vi "Relay test.vi"() -> ()   [LabVIEW 2021]
uses:
  ELAN/enums/main_prog_state.ctl
  ELAN/enums/init_state.ctl
  Master CR.lvclass
  Param/TCP Param/TCP Param.lvclass
  D:/my_projects/projects/21/Master CR/Param/Param.lvclass
  Master CR.lvclass/Master CR.ctl
  Param/Param.lvclass/Param.ctl
  Param/TCP Param/TCP Param.lvclass/TCP Param.ctl
  <vilib>/Platform/TimedLoop/XDataNode/timing_clust.ctl
  <vilib>/Platform/TimedLoop/XDataNode/nitl_modes.ctl
  <vilib>/Platform/TimedLoop/XDataNode/wakeup.ctl
  ELAN/enums/close_state.ctl
  Data/Data Model/Read Data Model.vi
  <vilib>/Utility/config.llb/Read Key (String).vi
  <vilib>/Utility/config.llb/Write Key (String).vi
  <vilib>/Platform/TimedLoop/XDataNode/XDataNode.xnode
  Modbus_v121c/Data Model/Device Data Model.lvclass
  <vilib>/Platform/TimedLoop/XDataNode/XDNodeRunTimeDep.lvlib
  ELAN/enums/Param_MB test.lvlib
  Param/Param.lvclass
  <vilib>/Utility/config.llb/NI_LVConfig.lvlib
panel:
  out "N2":u64
  out "N1":u64
  in  "Write":bool
  in  "Read":bool
  out "connects":bool[](array[boolean])
  out "DI":bool[](array[boolean])
  in  "DO":bool[](array[boolean])
  in  "AOint":u16[](array[numeric])
  out "comm error":errorcluster
  out "initialise error":errorcluster
  in  "EP_on":bool
  in  "tick":i64=1000 caption="Время цикла основной программы" min=5 max=2000 step=1
  in  "stop":bool
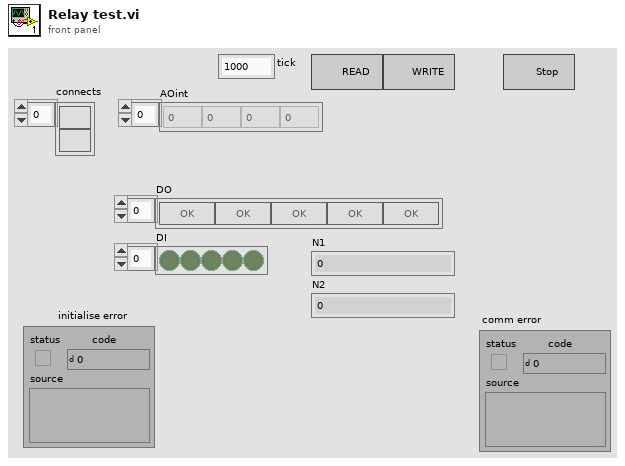
[diagram p1: front panel]
types:
  T1 = cluster{"conn_timeout":i32, "reconn_timeout":i32, "N attempt max":i32, "t_reset_TTL":i32, "write_timeout":i32, "read_timeout":i32, "period":i32}[]
  T2 = cluster{"Remote IP Address":string, "Remote Port":u16}[]
  T3 = typedef "Param_MB test.lvlib/init_state.ctl" = enum16{"Init Data", "Init TMPs", "Init system DB", "Init data DB", "Read Enums", "Init arrays", "Init KFM", "Init Param", "Init AI param", "Init DI param", "Init AO param", "Init DO param", "Init ALR param", "Init save progs", "Read OPC param", "Init Shared Variables", "Init regulators", "Init heaters", "Init Y defs", "Exit"}
  T4 = typedef "Param_MB test.lvlib/main_prog_state.ctl" = enum16{"Read_AI_Param", "Read_DI_Param", "Read_AO_Param", "Read_DO_Param", "Read_ALR_ON_OFF", "Read_ALR_Param", "Read_Param", "Read_REG_Param", "Timers", "AI", "DI", "SendAItoScada", "SendDItoScada", "Alarms", "SendAItoDB", "SendDItoDB", "SendALRtoDB", "Messages", "Controls", "Control HT1", "QN_control", "QN", "QN_state", "Control EB3", "Outputs", "Exit"}
  T5 = cluster{"KFM":string[], "PAR":string[], "AI":string[], "DI":string[], "DI_fast":string[], "AO":string[], "Regs":string[], "DO":string[], "ALR":string[], "System":string[]}
  T6 = typedef "NI_LVConfig.lvlib/Config Data RefNum.ctl" = refnum<k1>
  T7 = cluster{"Enums":cluster{"KFM":string[], "PAR":string[], "AI":string[], "DI":string[], "DI_fast":string[], "AO":string[], "Regs":string[], "DO":string[], "ALR":string[], "System":string[]}, "MBs":refnum<class "Master CR.lvclass">[], "N":string[]}
  T8 = cluster{"current time":timestamp, "Timer_1s":bool, "Timer_10s":bool, "Timer_1day":bool}
  T9 = typedef "XDNodeRunTimeDep.lvlib/timing_clust.ctl" = cluster{"Expected End [f-1]":u64, "Actual End [f-1]":u64, "Finished Late? [f-1]":bool, "Expected End [i-1]":u64, "Actual End [i-1]":u64, "Finished Late? [i-1]":bool, "Expected Start [i]":u64, "Actual Start [i]":u64, "Expected Start [f]":u64, "Actual Start [f]":u64, "Source Name":string, "Structure Name":string, "Period":i64, "Deadline":i64, "Offset":i64, "Start":i64, "Priority":i32, "Timeout":i32, "Mode":T10, "Wakeup Reason":T11, "Error":errorcluster, "Source Type":string, "Secondary Source Type":string, "Global End Time":u64, "Global Start Time":u64, "Frame Duration":u64, "Iteration Duration":u64, "Assigned CPU":i32, "I/O Scan Engine Mode":u32}
  T10 = typedef "XDNodeRunTimeDep.lvlib/nitl_modes.ctl" = enum32{"No Change", "Process missed periods, maintain original phase", "Discard missed periods, maintain original phase", "Process missed periods, ignore original phase", "Discard missed periods, ignore original phase"}
  T11 = typedef "XDNodeRunTimeDep.lvlib/wakeup.ctl" = enum32{"Normal", "Aborted", "Asynchronous wakeup", "Timing source error", "Timed loop error", "Timeout"}
  T12 = typedef "Param_MB test.lvlib/close_state.ctl" = enum16{"QN_state notifier", "QN_control_queue", "ALR notifires", "ALR", "DO notifires", "DO", "AO notifires", "AO", "DI notifres", "DI", "AI notifires", "AI", "OPC", "Param", "SaveMessageProg", "KFM DadaRef", "KFM Registers", "KFM StatusRef", "Exit"}
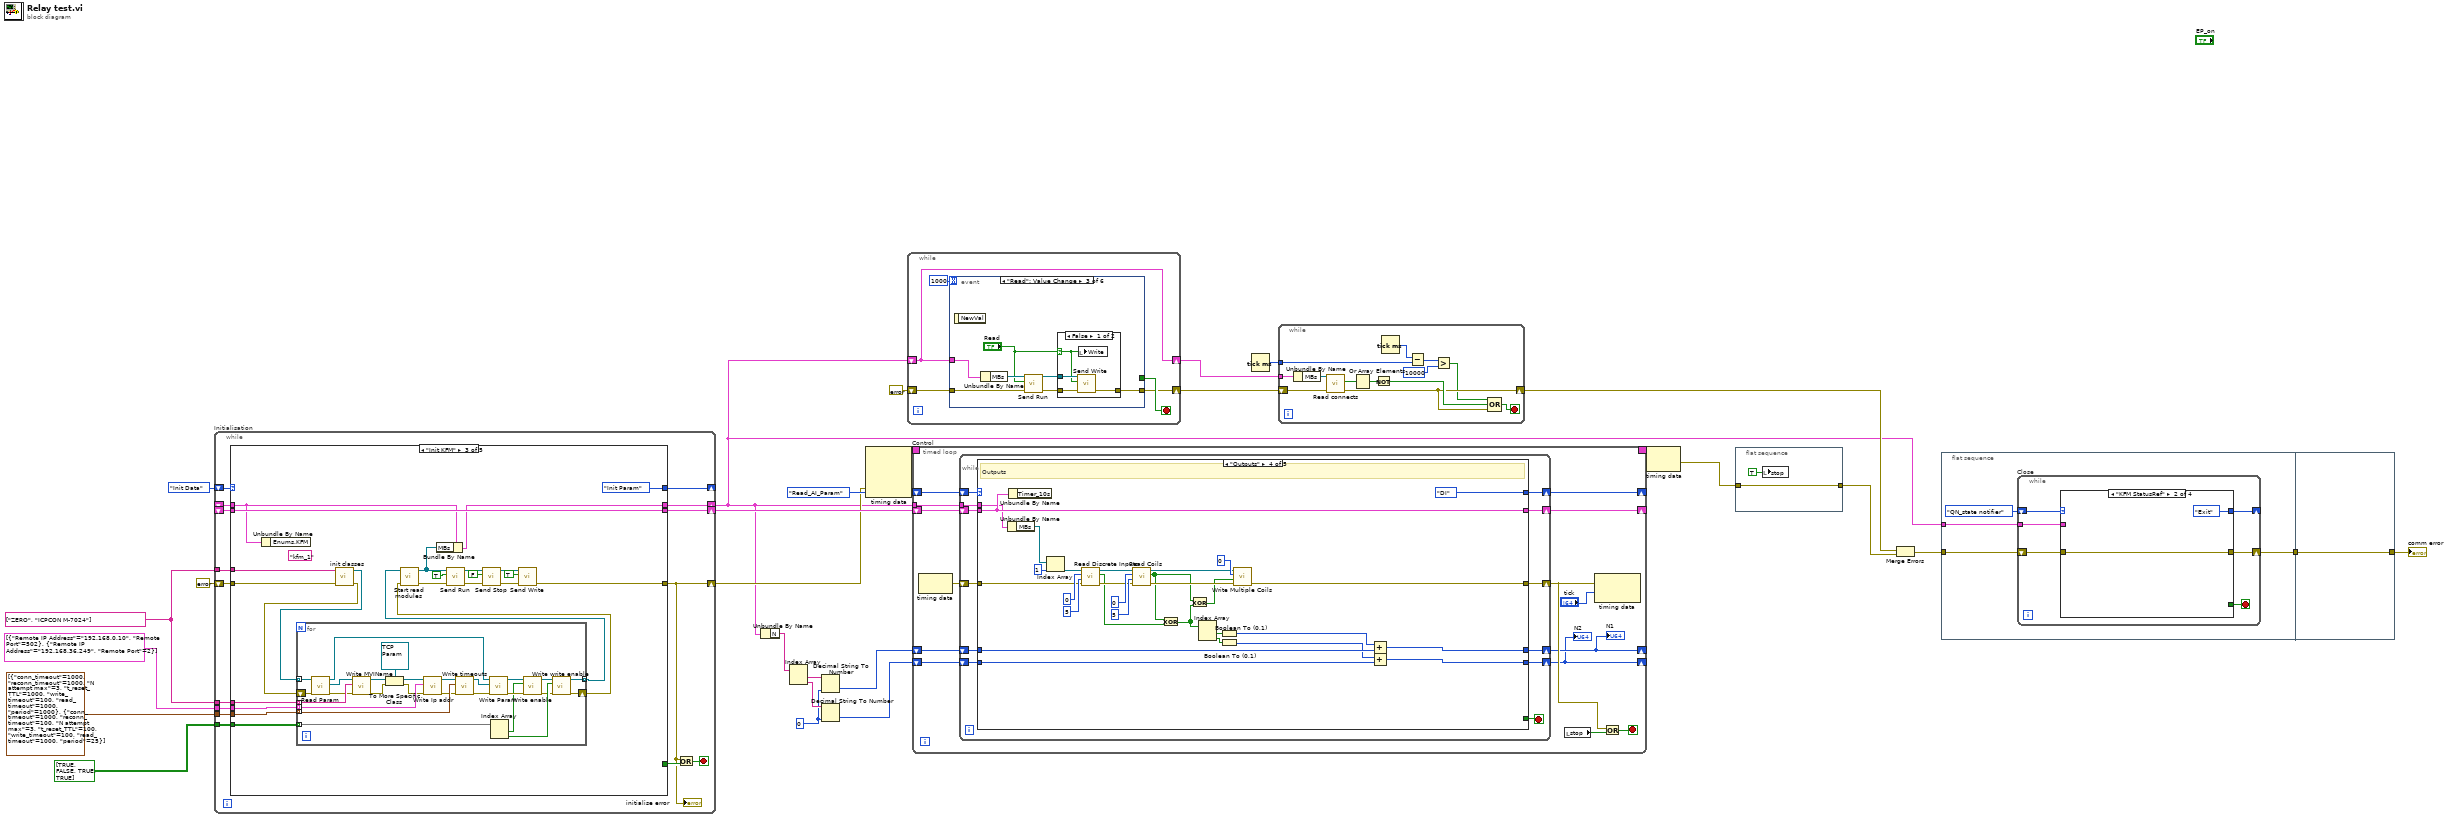
[diagram p0: block diagram]
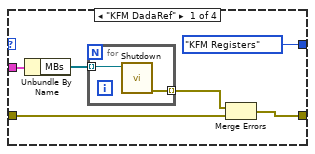
[diagram p2: hidden frame]
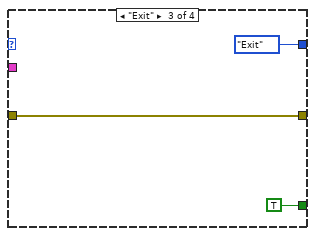
[diagram p3: hidden frame]
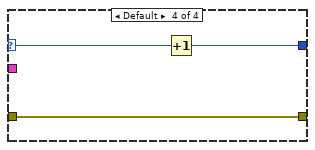
[diagram p4: hidden frame]
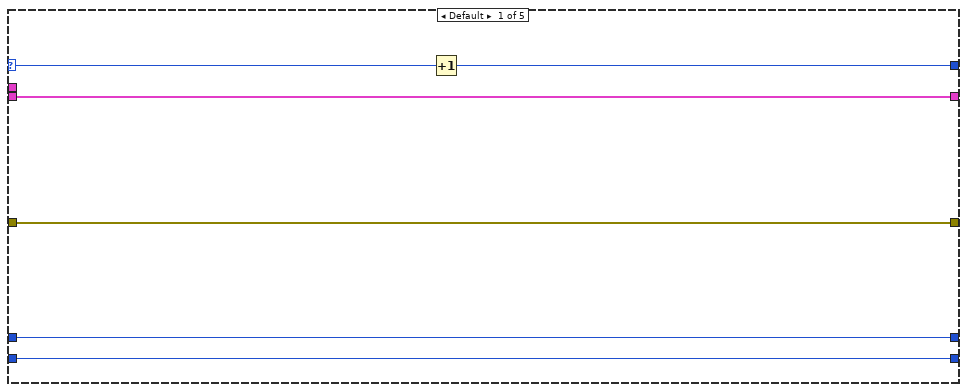
[diagram p5: hidden frame]
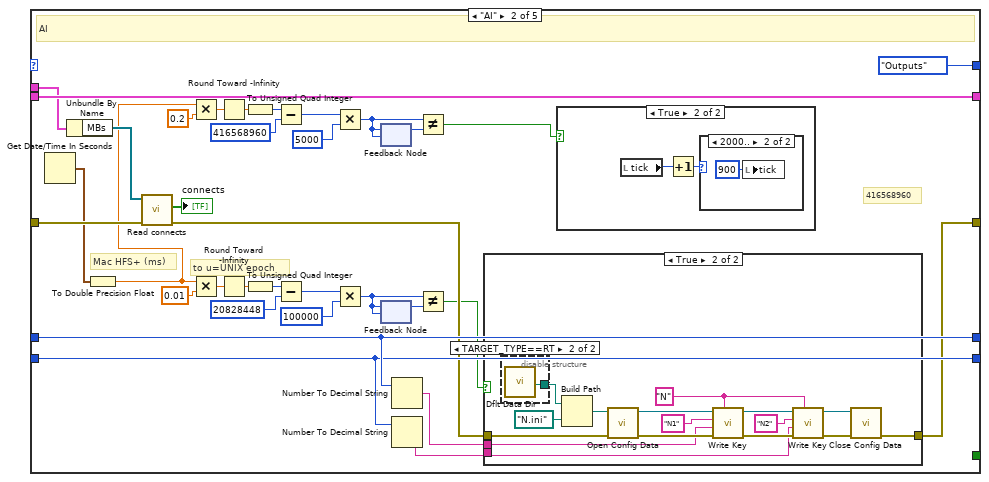
[diagram p6: hidden frame]
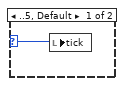
[diagram p8: hidden frame]
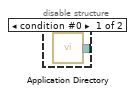
[diagram p10: hidden frame]
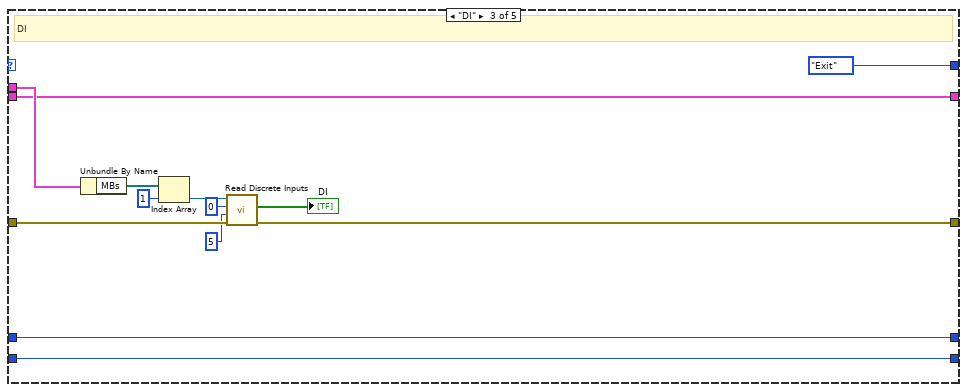
[diagram p11: hidden frame]
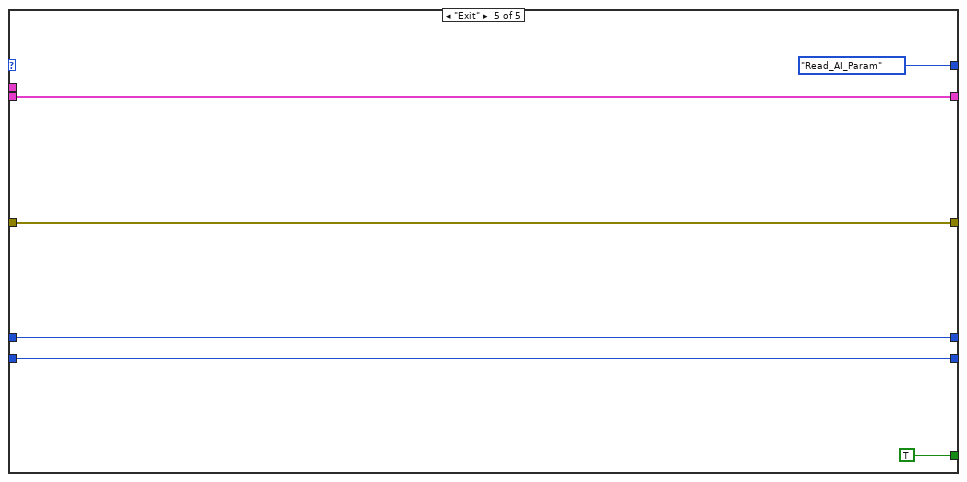
[diagram p12: hidden frame]
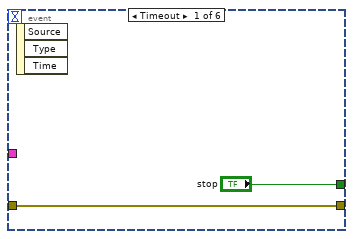
[diagram p13: hidden frame]
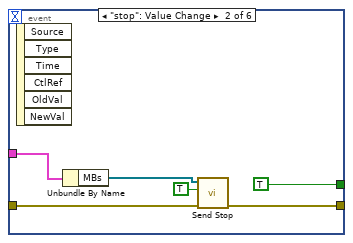
[diagram p14: hidden frame]
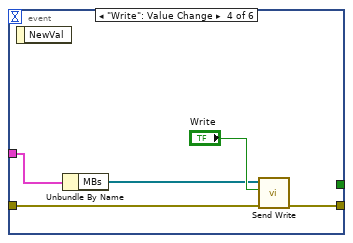
[diagram p16: hidden frame]
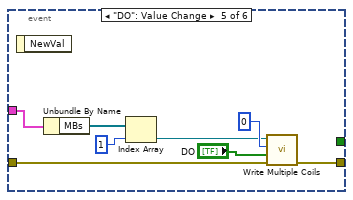
[diagram p17: hidden frame]
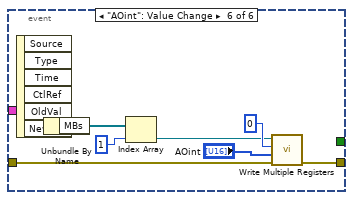
[diagram p18: hidden frame]
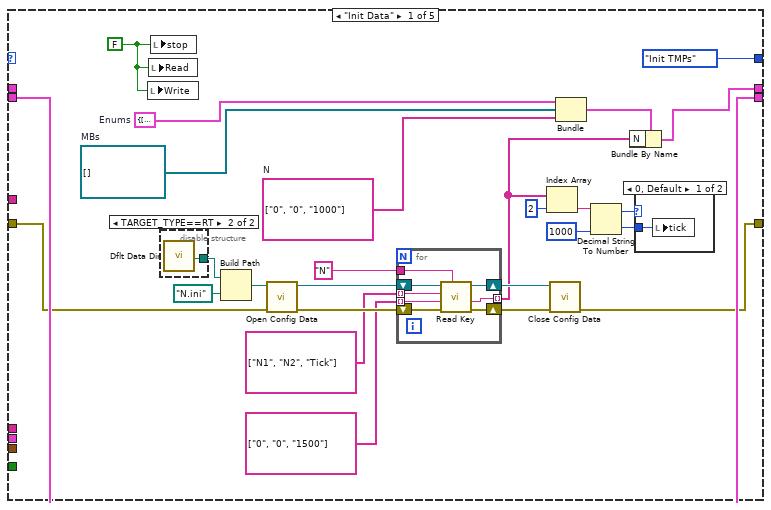
[diagram p19: hidden frame]
diagram:
  w3 = u64 0
  w15 = string[] ["ZERO", "ICPCON M-7024"] ("MVIName")
  n1 = while "Initialisation" {
    shift-right: [w34] -> w14
    shift-left: errorcluster {"status"=FALSE, "code"=0, "source"=""} ("error out") -> [w40]
    shift-right: [w43] -> w7
    shift-left: _ -> [w41]
    shift-right: [w39] -> _
    shift-left: init_state."Init Data" -> [w42]
    shift-right: [w36] -> w22
    shift-left: _ -> [w35]
    tunnel: w15 -> [w33]
    tunnel: T2 [{"Remote IP Address"="192.168.0.10", "Remote Port"=502}, {"Remote IP Address"="192.168.36.249", "Remote Port"=2}] ("IP Address") -> [w32]
    tunnel: T1 [{"conn_timeout"=1000, "reconn_timeout"=1000, "N attempt max"=3, "t_reset_TTL"=1000, "write_timeout"=100, "read_timeout"=1000, "period"=1000}, {"conn_timeout"=1000, "reconn_timeout"=100, "N attempt max"=3, "t_reset_TTL"=100, "write_timeout"=100, "read_timeout"=1000, "period"=25}] ("timeouts") -> [w31]
    tunnel: bool[][] [[TRUE, FALSE], [TRUE, TRUE]] ("enable") -> [w30]
    tunnel: w15 -> [w29]
    stop <- w37 stop-if-true
    # "Initialisation"
    n2 = case shown="\"Init KFM\"" w42 {
      tunnel: [w54 w87 w91 w141 w144] -> w34
      selector: w42 -> [_ _ _ _ w147]
      tunnel: [w50 w86 w93 w142 w145] -> w43
      tunnel: w41 -> [_ w86 w110 w142 w145]
      tunnel: w40 -> [w53 w87 w109 w141 w144]
      tunnel: [init_state."Init TMPs" init_state."Init system DB" init_state."Init Param" init_state."Init Data" w146] -> w39
      tunnel: [_ _ _ TRUE _] -> w38
      tunnel: [w67 w85 w111 w139 w148] -> w36
      tunnel: w35 -> [w67 _ w111 w139 w148]
      tunnel: w33 -> [_ _ w104 _ _]
      tunnel: w32 -> [_ _ w103 _ _]
      tunnel: w31 -> [_ _ w102 _ _]
      tunnel: w30 -> [_ _ w101 _ _]
      tunnel: w29 -> [_ _ w100 _ _]
      frame "Init Data" {
        w52 = string[] ["0", "0", "1000"]  # N
        w65 = FALSE ("stop")
        w66 = refnum<class "Master CR.lvclass">[] []  # MBs
        w68 = T5 {"KFM"=[], "PAR"=[], "AI"=[], "DI"=[], "DI_fast"=[], "AO"=[], "Regs"=[], "DO"=[], "ALR"=[], "System"=[]}  # Enums
        n3 = local write "Write"(w65) -> ()
        n4 = local write "Read"(w65) -> ()
        n5 = local write "stop"(w65) -> ()
        n6 = disable-structure shown="TARGET_TYPE==RT" {
          disable-tunnel: [w79 w80] -> w60
          frame condition #0 {
            n7 = call <vilib>:"Application Directory.vi"() -> ("Application Directory"=w79:path)
          }
          frame condition #1 (active) {
            n8 = call <vilib>:"Dflt Data Dir.vi"() -> ("App:Default Data Directory"=w80:path)
          }
        }
        n9 = Build Path(base path=w60, name or relative path=path "N.ini" ("configuration file path")) -> (appended path=w64:path)
        n10 = call <vilib>:"Open Config Data.vi"("error in (no error)"=w53, "configuration file path"=w64) -> ("error out"=w63:errorcluster, "refnum"=w62:T6)  [unwired: 7 in, 1 out]
        n11 = for {
          tunnel: "N" ("key") -> [w75]
          shift-right: [w73] -> w58
          shift-left: w63 -> [w78]
          shift-right: [w72] -> w57
          shift-left: w62 -> [w77]
          tunnel: string[] ["N1", "N2", "Tick"] -> [w76] mode=indexing
          tunnel: [w74] -> w49 mode=indexing
          tunnel: string[] ["0", "0", "1500"] -> [w71] mode=indexing
          n12 = call-poly <vilib>:"Read Key.vi"("section"=w75, "error in (no error)"=w78, "default value"=w71, "key"=w76, "refnum"=w77) -> ("error out"=w73:errorcluster, "value"=w74:string, "refnum out"=w72:T6)  [unwired: 3 in, 1 out]
        }
        n13 = Index Array(array=w49, index=2) -> (element=w46:string)
        n14 = call <vilib>:"Close Config Data.vi"("error in (no error)"=w58, "refnum"=w57) -> ("error out"=w54:errorcluster)  [unwired: 8 in, 1 out]
        n15 = Bundle("Enums"=w68, "MBs"=w66, "N"=w52) -> (w51:T7)  [unwired: 1 in]
        n16 = Decimal String To Number(string=w46, default (0L)=i64 1000 ("tick")) -> (offset past number=w45:i32, number=w44:i64)  [unwired: 1 in]
        n17 = Bundle By Name(cluster=w51, "N"=w49) -> (w50:T7)
        n18 = case shown="0, Default" w45 {
          tunnel: w44 -> [w70 _]
          frame 0, Default {
            n19 = local write "tick"(w70) -> ()
          }
          frame -1 {
          }
        }
      }
      frame "Init TMPs" {
        w81 = FALSE  # Timer_10s
        w82 = FALSE  # Timer_1day
        w83 = FALSE  # Timer_1s
        w84 = timestamp(0 s since 1904-01-01)  # current time
        n20 = Bundle("current time"=w84, "Timer_1s"=w83, "Timer_10s"=w81, "Timer_1day"=w82) -> (w85:T8)  [unwired: 1 in]
      }
      frame "Init KFM" {
        (unwired) "kfm_1" ("KFMTable")
        n21 = Unbundle By Name(w110) -> ()  [unwired: 1 out]
        n22 = call "init classes.vi"("error in (no error)"=w109, "MVINames"=w100) -> ("error out"=w106:errorcluster, "MBs"=w108:refnum<class "Master CR.lvclass">[])  [unwired: 8 in]
        n23 = for {
          tunnel: w108 -> [w114] mode=indexing
          tunnel: w103 -> [w121] mode=indexing
          tunnel: w102 -> [w118] mode=indexing
          tunnel: w104 -> [w136] mode=indexing
          tunnel: w101 -> [w130] mode=indexing
          tunnel: [w126] -> w107 mode=indexing
          shift-right: [w125] -> w105
          shift-left: w106 -> [w138]
          n24 = call "Read Param.vi"("error in (no error)"=w138, "MB_TCP in"=w114) -> ("error out"=w134:errorcluster, "Param"=w113:refnum<class "Param.lvclass">, "MB_TCP out"=w133:refnum<class "Master CR.lvclass">)  [unwired: 7 in]
          n25 = call "Write MVIName.vi"("error in (no error)"=w134, "MVIName"=w136, "MB Param in"=w113) -> ("error out"=w123:errorcluster, "MB Param out"=w135:refnum<class "Param.lvclass">)  [unwired: 7 in]
          n26 = To More Specific Class(target class=refnum<class "TCP Param.lvclass"> refnum ("Param.lvlib:TCP Param.lvclass"), reference=w135, error in=w123) -> (specific class reference=w122:refnum<class "TCP Param.lvclass">, error out=w120:errorcluster)
          n27 = call "Write Ip addr.vi"("error in (no error)"=w120, "IP address"=w121, "MB Param in"=w122) -> ("error out"=w117:errorcluster, "MB Param out"=w119:refnum<class "TCP Param.lvclass">)  [unwired: 7 in]
          n28 = call "Write timeouts.vi"("error in (no error)"=w117, "timeouts"=w118, "MB Param in"=w119) -> ("error out"=w116:errorcluster, "MB Param out"=w115:refnum<class "TCP Param.lvclass">)  [unwired: 7 in]
          n29 = call "Write Param.vi"("error in (no error)"=w116, "Param"=w115, "MB_TCP in"=w133) -> ("error out"=w131:errorcluster, "MB_TCP out"=w132:refnum<class "Master CR.lvclass">)  [unwired: 7 in]
          n30 = Index Array(array=w130) -> (element #1=w129:bool, element #2=w128:bool)  [unwired: 2 in]
          n31 = call "Write enable.vi"("error in (no error)"=w131, "enable"=w129, "Master CR in"=w132) -> ("error out"=w127:errorcluster, "Master CR out"=w137:refnum<class "Master CR.lvclass">)  [unwired: 7 in]
          n32 = call "Write write enable.vi"("error in (no error)"=w127, "write enable"=w128, "Master CR in"=w137) -> ("error out"=w125:errorcluster, "Master CR out"=w126:refnum<class "Master CR.lvclass">)  [unwired: 7 in]
        }
        n33 = call "Start read modules.vi"("error in"=w105, "classes"=w107) -> ("error out"=w95:errorcluster, "classes initialised"=w94:refnum<class "Master CR.lvclass">[])  [unwired: 8 in]
        n34 = Bundle By Name(cluster=w110, "MBs"=w94) -> (w93:T7)
        n35 = call "Send Run.vi"("error in"=w95, "Run"=TRUE, "MCRs"=w94) -> ("error out"=w98:errorcluster, "MCRs out"=w99:refnum<class "Master CR.lvclass">[])  [unwired: 7 in]
        n36 = call "Send Stop.vi"("error in"=w98, "Stop"=FALSE ("Write"), "MCRs"=w99) -> ("error out"=w92:errorcluster, "MCRs out"=w90:refnum<class "Master CR.lvclass">[])  [unwired: 7 in]
        n37 = call "Send Write.vi"("error in"=w92, "Write"=TRUE, "MCRs"=w90) -> ("error out"=w91:errorcluster)  [unwired: 7 in, 1 out]
      }
      frame "Exit" {
      }
      frame Default {
        n38 = Increment(x=w147) -> (x+1=w146:T3)
      }
    }
    "initialise error" <- w34
    n39 = Or(x=w34, y=w38) -> (x .or. y?=w37:bool)
  }
  n40 = Unbundle By Name(w7) -> ("N"=w6:string[])
  n41 = Index Array(array=w6) -> (element #1=w5:string, element #2=w4:string)  [unwired: 2 in]
  n42 = Decimal String To Number(string=w5, default (0L)=w3) -> (number=w2:u64)  [unwired: 1 in, 1 out]
  n43 = Decimal String To Number(string=w4, default (0L)=w3) -> (number=w1:u64)  [unwired: 1 in, 1 out]
  n44 = node-c288(w14) -> (w28:T9)  [unwired: 3 in]
  n45 = while {
    shift-right: [w151] -> w11
    shift-left: errorcluster {"status"=FALSE, "code"=0, "source"=""} ("error out") -> [w150]
    shift-right: [w149] -> w10
    shift-left: w7 -> [w149]
    stop <- w152 stop-if-true
    n46 = event shown="[2] \"Read\": Value Change" {
      selector: _ -> [_ _ _ _ _ _]
      dyn-events: _ -> [_ _ _ _ _ _]
      timeout: 1000 -> [_ _ _ _ _ _]
      tunnel: ["stop" TRUE ("stop") _ _ _ _] -> w152
      tunnel: w149 -> [_ w156 w168 w178 w186 w194]
      tunnel: w150 -> [w154 w160 w167 w177 w183 w189]
      tunnel: [w154 w159 w162 w176 w182 w188] -> w151
      event Timeout {
        n47 = event-data() -> ()  [unwired: 1 in, 3 out]
      }
      event "stop": Value Change {
        n48 = event-data() -> ()  [unwired: 1 in, 6 out]
        n49 = Unbundle By Name(w156) -> ("MBs"=w157:refnum<class "Master CR.lvclass">[])
        n50 = call "Send Stop.vi"("error in"=w160, "Stop"=TRUE, "MCRs"=w157) -> ("error out"=w159:errorcluster)  [unwired: 7 in, 1 out]
      }
      event "Read": Value Change {
        n51 = event-data() -> ()  [unwired: 1 in, 1 out]
        n52 = Unbundle By Name(w168) -> ("MBs"=w166:refnum<class "Master CR.lvclass">[])
        n53 = call "Send Run.vi"("error in"=w167, "Run"="Read", "MCRs"=w166) -> ("error out"=w164:errorcluster, "MCRs out"=w163:refnum<class "Master CR.lvclass">[])  [unwired: 7 in]
        n54 = case shown="False" "Read" {
          selector: "Read" -> [w170 _]
          tunnel: w164 -> [w172 w173]
          tunnel: w163 -> [w171 _]
          tunnel: [w169 w173] -> w162
          frame False {
            n55 = call "Send Write.vi"("error in"=w172, "Write"=w170, "MCRs"=w171) -> ("error out"=w169:errorcluster)  [unwired: 7 in, 1 out]
            n56 = local write "Write"(w170) -> ()
          }
          frame True {
          }
        }
      }
      event "Write": Value Change {
        n57 = event-data() -> ()  [unwired: 1 in, 1 out]
        n58 = Unbundle By Name(w178) -> ("MBs"=w174:refnum<class "Master CR.lvclass">[])
        n59 = call "Send Write.vi"("error in"=w177, "Write"="Write", "MCRs"=w174) -> ("error out"=w176:errorcluster)  [unwired: 7 in, 1 out]
      }
      event "DO": Value Change {
        n60 = event-data() -> ()  [unwired: 1 in, 1 out]
        n61 = Unbundle By Name(w186) -> ("MBs"=w180:refnum<class "Master CR.lvclass">[])
        n62 = Index Array(array=w180, index=1) -> (element=w179:refnum<class "Master CR.lvclass">)
        n63 = call-dynamic "Write Multiple Coils.vi"("error in"=w183, "coils"="DO", "starting address"=u16 0, "Master CR in"=w179) -> ("error out"=w182:errorcluster)  [unwired: 6 in, 1 out]
      }
      event "AOint": Value Change {
        n64 = event-data() -> ()  [unwired: 1 in, 6 out]
        n65 = Unbundle By Name(w194) -> ("MBs"=w192:refnum<class "Master CR.lvclass">[])
        n66 = Index Array(array=w192, index=1) -> (element=w187:refnum<class "Master CR.lvclass">)
        n67 = call-dynamic "Write Multiple Registers.vi"("error in"=w189, "register values"="AOint", "starting address"=u16 0, "Master CR in"=w187) -> ("error out"=w188:errorcluster)  [unwired: 6 in, 1 out]
      }
    }
  }
  n68 = timed-loop "Control" {
    tunnel: w7 -> [w208]
    shift-right: [w206] -> _
    shift-left: w22 -> [w207]
    timing: w28 -> [_]
    timing-out: [_] -> w27
    shift-right: [w204] -> _
    shift-left: main_prog_state."Read_AI_Param" -> [w203]
    shift-right: [w198] -> _
    shift-left: w2 -> [w197]
    shift-right: [w195] -> _
    shift-left: w1 -> [w196]
    stop <- w201 stop-if-true
    n69 = node-c288() -> (w205:errorcluster)  [unwired: 1 in]
    n70 = while {
      tunnel: w208 -> [w220]
      shift-right: [w218] -> w206
      shift-left: w207 -> [w219]
      shift-right: [w213] -> w199
      shift-left: w205 -> [w217]
      shift-right: [w216] -> w204
      shift-left: w203 -> [w215]
      shift-right: [w212] -> w198
      shift-left: w197 -> [w210]
      shift-right: [w211] -> w195
      shift-left: w196 -> [w209]
      stop <- w214 stop-if-true
      n71 = case shown="\"Outputs\"" w215 {
        tunnel: w217 -> [w223 w259 w293 w314 w328]
        tunnel: w220 -> [_ w256 w295 w323 _]
        tunnel: w219 -> [w225 w258 w294 w324 w329]
        tunnel: [w225 w258 w294 w324 w329] -> w218
        selector: w215 -> [w226 _ _ _ _]
        tunnel: [w224 main_prog_state."Outputs" main_prog_state."Exit" main_prog_state."DI" main_prog_state."Read_AI_Param"] -> w216
        tunnel: [_ _ _ _ TRUE] -> w214
        tunnel: [w223 w242 w291 w322 w328] -> w213
        tunnel: [w222 w245 w285 w302 w327] -> w212
        tunnel: [w221 w244 w284 w299 w326] -> w211
        tunnel: w210 -> [w222 w245 w285 w301 w327]
        tunnel: w209 -> [w221 w244 w284 w300 w326]
        frame Default {
          n72 = Increment(x=w226) -> (x+1=w224:T4)
        }
        frame "AI" {
          # "416568960"
          # "to u=UNIX epoch"
          # "Mac HFS+ (ms)"
          # "AI"
          n73 = Get Date/Time In Seconds() -> (seconds since 1Jan1904=w238:timestamp)
          n74 = Unbundle By Name(w256) -> ("MBs"=w255:refnum<class "Master CR.lvclass">[])
          n75 = To Double Precision Float(number=w238) -> (double precision float=w228:dbl)
          n76 = call "Read connects.vi"("error in (no error)"=w259, "MCRs in"=w255) -> ("error out"=w243:errorcluster, "connects"=→"connects":bool[])  [unwired: 7 in, 1 out]
          n77 = Multiply(x=w228, y=0.2) -> (x*y=w236:dbl)
          n78 = Multiply(x=w228, y=0.01) -> (x*y=w247:dbl)
          n79 = Round Toward -Infinity(1:w236) -> (0:w237:dbl)
          n80 = Round Toward -Infinity(1:w247) -> (0:w246:dbl)
          n81 = To Unsigned Quad Integer(1:w237) -> (0:w234:u64)
          n82 = To Unsigned Quad Integer(1:w246) -> (0:w249:u64)
          n83 = Subtract(x=w234, y=u64 416568960) -> (x-y=w235:u64)
          n84 = Subtract(x=w249, y=u64 20828448) -> (x-y=w248:u64)
          n85 = Multiply(x=w235, y=u64 5000) -> (x*y=w229:u64)
          n86 = Multiply(x=w248, y=u64 100000) -> (x*y=w254:u64)
          n87 = feedback #1(w229) -> (w230:u64)
          n88 = feedback-in #1(w229) -> ()
          n89 = feedback #2(w254) -> (w253:u64)
          n90 = feedback-in #2(w254) -> ()
          n91 = Number To Decimal String(number=w245) -> (decimal integer string=w241:string)  [unwired: 1 in]
          n92 = Number To Decimal String(number=w244) -> (decimal integer string=w240:string)  [unwired: 1 in]
          n93 = Not Equal?(x=w229, y=w230) -> (x != y?=w227:bool)
          n94 = Not Equal?(x=w254, y=w253) -> (x != y?=w239:bool)
          n95 = case shown="True" w239 {
            tunnel: w243 -> [w265 w270]
            tunnel: [w265 w269] -> w242
            tunnel: w241 -> [_ w268]
            tunnel: w240 -> [_ w267]
            frame False {
            }
            frame True {
              w266 = "N" ("key")
              n96 = disable-structure shown="TARGET_TYPE==RT" {
                disable-tunnel: [w282 w283] -> w274
                frame condition #0 {
                  n97 = call <vilib>:"Application Directory.vi"() -> ("Application Directory"=w282:path)
                }
                frame condition #1 (active) {
                  n98 = call <vilib>:"Dflt Data Dir.vi"() -> ("App:Default Data Directory"=w283:path)
                }
              }
              n99 = Build Path(base path=w274, name or relative path=path "N.ini" ("configuration file path")) -> (appended path=w271:path)
              n100 = call <vilib>:"Open Config Data.vi"("error in (no error)"=w270, "configuration file path"=w271) -> ("error out"=w272:errorcluster, "refnum"=w273:T6)  [unwired: 7 in, 1 out]
              n101 = call-poly <vilib>:"Write Key.vi"("section"=w266, "error in (no error)"=w272, "value"=w268, "key"="N1", "refnum"=w273) -> ("error out"=w277:errorcluster, "refnum out"=w276:T6)  [unwired: 4 in, 1 out]
              n102 = call-poly <vilib>:"Write Key.vi"("section"=w266, "error in (no error)"=w277, "value"=w267, "key"="N2", "refnum"=w276) -> ("error out"=w281:errorcluster, "refnum out"=w280:T6)  [unwired: 4 in, 1 out]
              n103 = call <vilib>:"Close Config Data.vi"("error in (no error)"=w281, "refnum"=w280) -> ("error out"=w269:errorcluster)  [unwired: 8 in, 1 out]
            }
          }
          n104 = case shown="True" w227 {
            frame False {
            }
            frame True {
              n105 = local read "tick"() -> (w262:i64)
              n106 = Increment(x=w262) -> (x+1=w261:i64)
              n107 = case shown="2000.." w261 {
                selector: w261 -> [w263 _]
                frame ..5, Default {
                  n108 = local write "tick"(w263) -> ()
                }
                frame 2000.. {
                  n109 = local write "tick"(i64 900 ("tick")) -> ()
                }
              }
            }
          }
        }
        frame "DI" {
          # "DI"
          n110 = Unbundle By Name(w295) -> ("MBs"=w290:refnum<class "Master CR.lvclass">[])
          n111 = Index Array(array=w290, index=1) -> (element=w287:refnum<class "Master CR.lvclass">)
          n112 = call "Read Discrete Inputs.vi"("error in"=w293, "number of inputs"=u16 5 ("number of coils"), "starting address"=u16 0, "Master CR in"=w287) -> ("error out"=w291:errorcluster, "discrete inputs"=→"DI":bool[])  [unwired: 5 in, 1 out]
        }
        frame "Outputs" {
          # "Outputs"
          n113 = Unbundle By Name(w323) -> ("MBs"=w320:refnum<class "Master CR.lvclass">[])
          n114 = Unbundle By Name(w324) -> ()  [unwired: 1 out]
          n115 = Index Array(array=w320, index=1) -> (element=w313:refnum<class "Master CR.lvclass">)
          n116 = call "Read Discrete Inputs.vi"("error in"=w314, "number of inputs"=u16 5, "starting address"=u16 0, "Master CR in"=w313) -> ("error out"=w312:errorcluster, "discrete inputs"=w310:bool[], "Master CR out"=w311:refnum<class "Master CR.lvclass">)  [unwired: 5 in]
          n117 = call "Read Coils.vi"("error in"=w312, "number of inputs"=u16 5, "starting address"=u16 0, "Master CR in"=w311) -> ("error out"=w309:errorcluster, "coils"=w306:bool[], "Master CR out"=w308:refnum<class "Master CR.lvclass">)  [unwired: 5 in]
          n118 = Exclusive Or(1:w310, 2:w306) -> (0:w305:bool[])
          n119 = Exclusive Or(1:w305, 2:w306) -> (0:w307:bool[])
          n120 = Index Array(array=w305) -> (element #1=w304:bool, element #2=w303:bool)  [unwired: 2 in]
          n121 = Boolean To (0,1)(Boolean=w304) -> (0, 1=w298:i16)
          n122 = Boolean To (0,1)(Boolean=w303) -> (0, 1=w297:i16)
          n123 = call-dynamic "Write Multiple Coils.vi"("error in"=w309, "coils"=w307, "starting address"=u16 0, "Master CR in"=w308) -> ("error out"=w322:errorcluster)  [unwired: 6 in, 1 out]
          n124 = Add(x=w298, y=w301) -> (x+y=w302:u64)
          n125 = Add(x=w297, y=w300) -> (x+y=w299:u64)
        }
        frame "Exit" {
        }
      }
    }
    "N1" <- w198
    "N2" <- w195
    n126 = local read "stop"() -> (w200:bool)
    n127 = node-c288(w199, "tick") -> ()  [unwired: 1 out]
    n128 = Or(x=w199, y=w200) -> (x .or. y?=w201:bool)
  }
  n129 = Tick Count (ms)() -> (millisecond timer value=w9:u32)
  n130 = while {
    shift-right: [w343] -> w8
    shift-left: w11 -> [w350]
    tunnel: w10 -> [w347]
    tunnel: w9 -> [w341]
    stop <- w345 stop-if-true
    n131 = Unbundle By Name(w347) -> ("MBs"=w346:refnum<class "Master CR.lvclass">[])
    n132 = call "Read connects.vi"("error in (no error)"=w350, "MCRs in"=w346) -> ("error out"=w343:errorcluster, "connects"=w349:bool[])  [unwired: 7 in, 1 out]
    n133 = Or Array Elements(Boolean array=w349) -> (logical OR=w348:bool)
    n134 = Not(x=w348) -> (.not. x?=w344:bool)
    n135 = Tick Count (ms)() -> (millisecond timer value=w342:u32)
    n136 = Subtract(x=w342, y=w341) -> (x-y=w340:u32)
    n137 = Greater?(x=w340, y=u32 10000) -> (0:w338:bool)
    n138 = Compound Arithmetic op=OR(w338, w344, w343) -> (w345:bool)
  }
  n139 = node-c288(w27) -> (w13:errorcluster)
  n140 = flat-sequence {
    tunnel: [w351] -> w12
    tunnel: w13 -> [w351]
    frame #0 {
      n141 = local write "stop"(TRUE ("stop")) -> ()
    }
  }
  n142 = Merge Errors(w8, w12) -> (w21:errorcluster)
  n143 = flat-sequence {
    tunnel: w7 -> [w355]
    tunnel: w21 -> [w354]
    tunnel: [w353] -> w20
    tunnel: [w379] -> w25
    tunnel: w20 -> [w379]
    frame #0 {
      n144 = while "Close" {
        shift-right: [w361] -> _
        shift-left: close_state."QN_state notifier" ("Init_state") -> [w362]
        tunnel: w355 -> [w359]
        shift-right: [w357] -> w353
        shift-left: w354 -> [w358]
        stop <- w360 stop-if-true
        n145 = case shown="\"KFM StatusRef\"" w362 {
          selector: w362 -> [_ _ _ w378]
          tunnel: [close_state."KFM Registers" close_state."Exit" close_state."Exit" w377] -> w361
          tunnel: [_ _ TRUE _] -> w360
          tunnel: w359 -> [w368 _ _ _]
          tunnel: w358 -> [w366 w371 w374 w376]
          tunnel: [w365 w371 w374 w376] -> w357
          frame "KFM DadaRef" {
            n146 = Unbundle By Name(w368) -> ("MBs"=w364:refnum<class "Master CR.lvclass">[])
            n147 = for {
              tunnel: w364 -> [w370] mode=indexing
              tunnel: [w369] -> w363 mode=indexing
              n148 = call-dynamic "Shutdown.vi"("MB in"=w370) -> ("error out"=w369:errorcluster)  [unwired: 10 in]
            }
            n149 = Merge Errors(w363, w366) -> (w365:errorcluster)
          }
          frame "KFM StatusRef" {
          }
          frame "Exit" {
          }
          frame Default {
            n150 = Increment(x=w378) -> (x+1=w377:T12)
          }
        }
      }
    }
    frame #1 {
    }
  }
  "comm error" <- w25
